vi "GetObjectStatus.vi"(0 "reference in":refnum<class "G#Object.lvclass">, 2 "simple info (F)":bool, 5 "error in (no error)":errorcluster) -> (8 "full class name":string, 9 "# of users?":i32, 10 "all object names":string[](array[string]), 11 "last user":bool, 12 "# of objects":i32, 13 "class name":string, 14 "reference out":refnum<class "G#Object.lvclass">, 15 "not a refnum?":bool, 16 "object name":string, 17 "all refs out":refnum<class "G#Object.lvclass">[](array[class]), 18 "counter?":bool, 19 "error out":errorcluster)   [LabVIEW 2017, in "G#Object.lvclass"]
doc: "Returns information about the specified object. If simple info = true, only object info is return and not the arrays of objects.\n\nIf input reference is invalid, only information about the class is returned."
uses:
  G#Object.lvclass
  G#Object.lvclass/G#Object.ctl
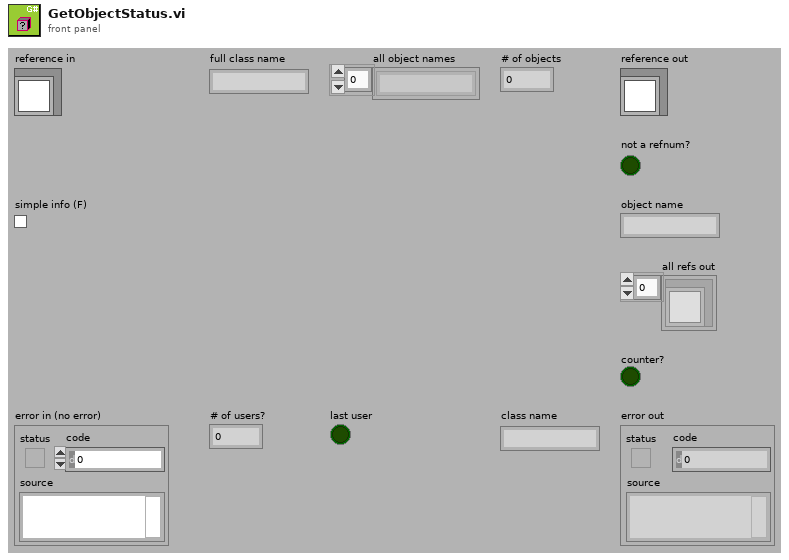
[diagram p1: front panel]
types:
  T1 = typedef "G#Object.lvclass/G#Object_ObjectInfoType.ctl" = cluster{"ObjectName":string, "ObjectID":u32, "Users":i32, "Counter":bool, "AttributeRefs":u32[], "FullClassName":string, "ClassName":string, "CreateMethod":T2, "GenericDestructorExists":bool, "Owner":string}
  T2 = typedef "G#Object.lvclass/G#Object_CreateMethod.ctl" = enum16{"Create", "Create or look up existing", "Look up existing"}
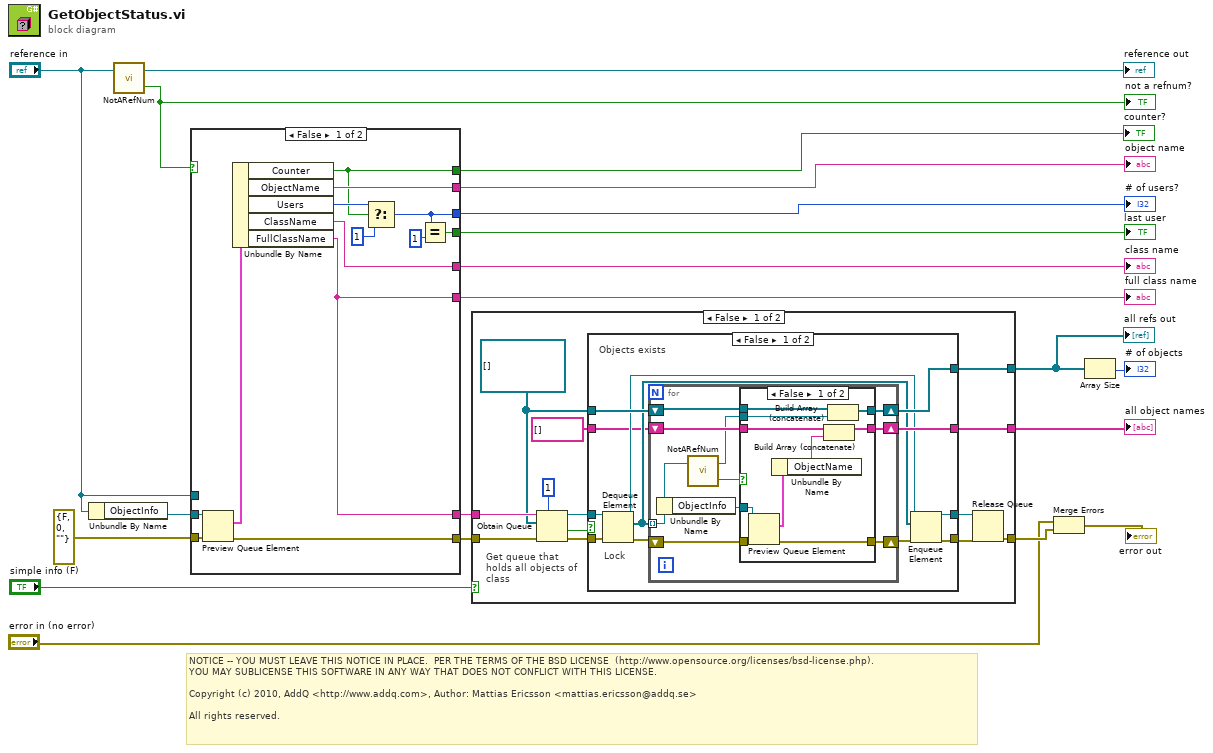
[diagram p0: block diagram]
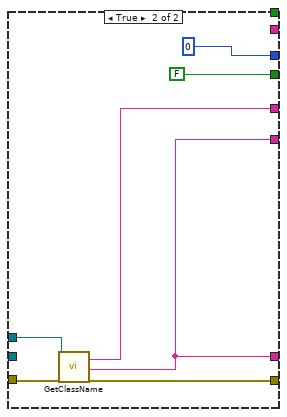
[diagram p5: hidden frame]
diagram:
  # "NOTICE -- YOU MUST LEAVE THIS NOTICE IN PLACE.  PER THE TERMS OF THE BSD LICENSE  (http://www.opensource.org/licenses/bsd-license.php).\nYOU MAY SUBLICENSE THIS SOFTWARE IN ANY WAY THAT DOES NOT CONFLICT WITH THIS LICENSE.\n\nCopyright (c) 2010, AddQ <http://www.addq.com>, Author: Mattias Ericsson <mattias.ericsson@addq.se>\n\nAll rights reserved."
  n1 = Unbundle By Name("reference in") -> ("ObjectInfo"=w20:refnum<queue>)
  n2 = call-dynamic "NotARefNum.vi"("reference in"="reference in") -> ("not a refnum?"=w1:bool, "reference out"=→"reference out":refnum<class "G#Object.lvclass">)  [unwired: 1 in]
  "not a refnum?" <- w1
  n3 = case shown="False" w1 {
    tunnel: errorcluster {"status"=FALSE, "code"=0, "source"=""} ("error in (no error)") -> [w33 w40]
    tunnel: w20 -> [w32 _]
    tunnel: [w30 _] -> w19
    tunnel: [w26 w35] -> w13
    tunnel: [w23 0 ("Users")] -> w18
    tunnel: [w28 FALSE] -> w17
    tunnel: [w27 w36] -> w16
    tunnel: "reference in" -> [_ w39]
    tunnel: [w25 w34] -> w12
    tunnel: [w22 _] -> w7
    tunnel: [w25 w34] -> w6
    frame False {
      n4 = Preview Queue Element(queue=w32, error in (no error)=w33) -> (element=w31:T1, error out=w26:errorcluster)  [unwired: 1 in, 2 out]
      n5 = Unbundle By Name(w31) -> ("Counter"=w22:bool, "ObjectName"=w30:string, "Users"=w24:i32, "ClassName"=w27:string, "FullClassName"=w25:string)
      n6 = Select(t=w24, s=w22, f=1) -> (s? t:f=w23:i32)
      n7 = Equal?(x=w23, y=1) -> (x = y?=w28:bool)
    }
    frame True {
      n8 = call-dynamic "GetClassName.vi"("reference in"=w39, "error in (no error)"=w40) -> ("class name"=w36:string, "full class name"=w34:string, "error out"=w35:errorcluster)  [unwired: 13 in, 2 out]
    }
  }
  "# of users?" <- w18
  "last user" <- w17
  "class name" <- w16
  "object name" <- w19
  "counter?" <- w7
  "full class name" <- w6
  n9 = case shown="False" "simple info (F)" {
    tunnel: w13 -> [w53 w91]
    tunnel: w12 -> [w52 _]
    tunnel: [w48 w91] -> w14
    tunnel: [w45 _] -> w9
    tunnel: [w43 _] -> w8
    frame False {
      w44 = refnum<class "G#Object.lvclass">[] [] ("element data type")
      # "Get queue that\nholds all objects of\nclass"
      n10 = Obtain Queue(max queue size (-1, unlimited)=1, name (unnamed)=w52, element data type=w44, error in (no error)=w53) -> (queue out=w47:refnum<queue>, created new?=w51:bool, error out=w50:errorcluster)  [unwired: 1 in]
      n11 = case shown="False" w51 {
        tunnel: w50 -> [w65 w90]
        tunnel: [w58 w90] -> w49
        tunnel: [w57 w89] -> w46
        tunnel: w47 -> [w64 w89]
        tunnel: [w60 _] -> w45
        tunnel: w44 -> [w62 _]
        tunnel: [w61 _] -> w43
        tunnel: string[] [] -> [w54 _]
        frame False {
          # "Lock"
          # "Objects exists"
          n12 = Dequeue Element(queue=w64, error in (no error)=w65) -> (queue out=w56:refnum<queue>, element=w55:refnum<class "G#Object.lvclass">[], error out=w63:errorcluster)  [unwired: 1 in, 1 out]
          n13 = for {
            shift-right: [w74] -> w59
            shift-left: w63 -> [w75]
            tunnel: w55 -> [w67] mode=indexing
            shift-right: [w69] -> w60
            shift-left: w62 -> [w70]
            shift-right: [w71] -> w61
            shift-left: w54 -> [w72]
            n14 = Unbundle By Name(w67) -> ("ObjectInfo"=w73:refnum<queue>)
            n15 = call-dynamic "NotARefNum.vi"("reference in"=w67) -> ("not a refnum?"=w68:bool, "reference out"=w66:refnum<class "G#Object.lvclass">)  [unwired: 1 in]
            n16 = case shown="False" w68 {
              tunnel: w75 -> [w85 w88]
              tunnel: [w84 w88] -> w74
              tunnel: w73 -> [w82 _]
              tunnel: w72 -> [w81 w86]
              tunnel: [w79 w86] -> w71
              tunnel: w70 -> [w78 w87]
              tunnel: w66 -> [w77 _]
              tunnel: [w76 w87] -> w69
              frame False {
                n17 = Preview Queue Element(queue=w82, error in (no error)=w85) -> (element=w83:T1, error out=w84:errorcluster)  [unwired: 1 in, 2 out]
                n18 = Unbundle By Name(w83) -> ("ObjectName"=w80:string)
                n19 = Build Array (concatenate)(w81, w80) -> (w79:string[])
                n20 = Build Array (concatenate)(w78, w77) -> (w76:refnum<class "G#Object.lvclass">[])
              }
              frame True {
              }
            }
          }
          n21 = Enqueue Element(queue=w56, element=w55, error in (no error)=w59) -> (queue out=w57:refnum<queue>, error out=w58:errorcluster)  [unwired: 1 in, 1 out]
        }
        frame True {
          # "No objects exists"
        }
      }
      n22 = Release Queue(queue=w46, error in (no error)=w49) -> (error out=w48:errorcluster)  [unwired: 1 in, 2 out]
    }
    frame True {
      # "Simple info -> Do not check all objects."
    }
  }
  "all refs out" <- w9
  "all object names" <- w8
  n23 = Merge Errors("error in (no error)", w14) -> (→"error out":errorcluster)
  n24 = Array Size(array=w9) -> (size(s)=→"# of objects":i32)
